vi "Test Process Cleared on Upstream Error.vi"(8 "error in (no error)":errorcluster, 11 "Process Test In":refnum<class "Process Dev Test.lvclass">) -> (0 "error out":errorcluster, 3 "Process Test Out":refnum<class "Process Dev Test.lvclass">)   [LabVIEW 2020, in "Process Dev Test.lvclass"]
uses:
  Process Dev Test.lvclass
  C:/Git/astemes-triarc-framework/source/TF Test Suite/Base Class Test/Base Test.lvclass
  C:/Program Files (x86)/National Instruments/LabVIEW 2020/vi.lib/Astemes/LUnit/Test Case.lvclass
  source/Framework/Process/Process.lvclass
  source/Framework/Process/Public/Lifecycle/Lifecycle State.ctl
  source/Framework Test Suite/Base Class Test/Base Test.lvclass/Base Test.ctl
  source/Framework/Process/Process.lvclass/Process.ctl
  <vilib>/Astemes/LUnit/Test Case.lvclass/Test Case.ctl
  <vilib>/Astemes/LUnit/LUnit Assertion Result.lvclass/LUnit Assertion Result.ctl
  <vilib>/Astemes/LUnit/LUnit Test Case Result.lvclass/LUnit Test Case Result.ctl
  <vilib>/Astemes/LUnit/LUnit Method Result.lvclass/LUnit Method Result.ctl
  <vilib>/Astemes/LUnit/Palette/Fail.vi
  <vilib>/Astemes/LUnit/Palette/Pass.vi
  <vilib>/Astemes/LUnit/Set Assertion Type.vi
  <vilib>/Astemes/LUnit/Add test result.vi
  <vilib>/Astemes/LUnit/LUnit Write Passed.vi
  <vilib>/Astemes/LUnit/LUnit Write Message.vi
  <vilib>/Astemes/LUnit/LUnit Write Description.vi
  <vilib>/Astemes/LUnit/LUnit Write Assertion Type.vi
  <vilib>/Astemes/LUnit/LUnit Record Assertion Result.vi
  <vilib>/Astemes/LUnit/LUnit Aggregate Assertion Results.vi
  <vilib>/Astemes/LUnit/Assertion Result/LUnit Read Status.vi
  <vilib>/Astemes/LUnit/LUnit Read Message.vi
  <vilib>/Astemes/LUnit/LUnit Read Description.vi
  <vilib>/Astemes/LUnit/Method Result/LUnit Merge Status.vi
  <vilib>/Astemes/LUnit/LUnit Concatenate result strings.vi
  source/Framework/Base/Base.lvclass
  <vilib>/Astemes/LUnit/LUnit Assertion Result.lvclass
  source/Framework Test Suite/Base Class Test/Base Test.lvclass
  <vilib>/Astemes/LUnit/Test Case.lvclass
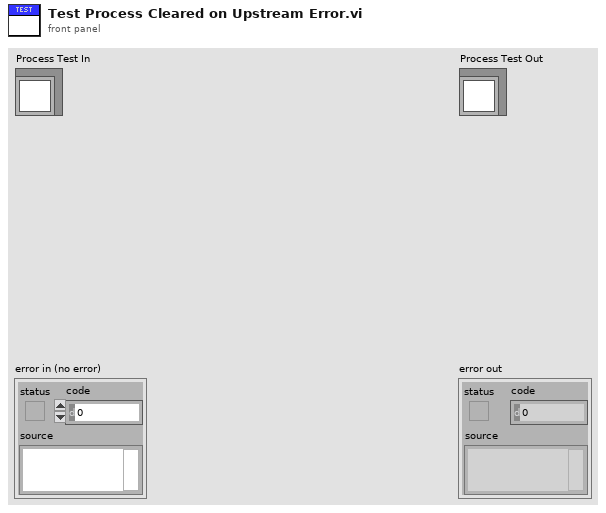
[diagram p1: front panel]
types:
  T1 = typedef "Process.lvclass/Lifecycle State.ctl" = enum16{"Uninitialized", "Initialized", "Started", "Running", "Stopped", "Finished"}
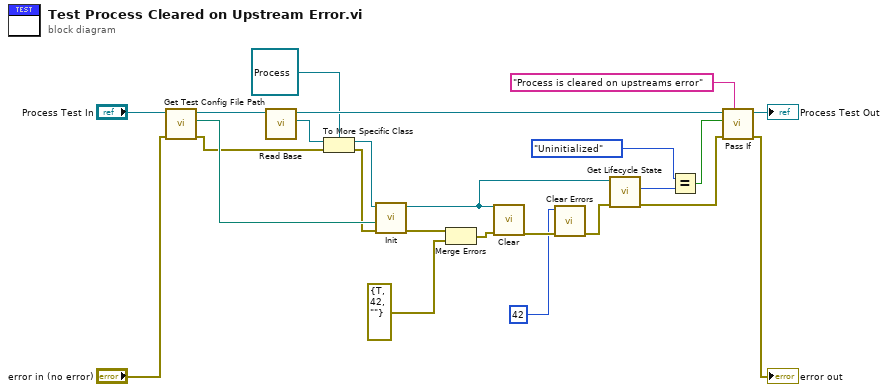
[diagram p0: block diagram]
diagram:
  n1 = call "Get Test Config File Path.vi"("error in (no error)"="error in (no error)", "Process Test In"="Process Test In") -> ("error out"=w14:errorcluster, "Test config path"=w20:path, "Process Test Out"=w22:refnum<class "Process Dev Test.lvclass">)  [unwired: 7 in]
  n2 = call "Read Base.vi"("Base Class Test In"=w22) -> ("Base.lvclass"=w17:refnum<class "Base.lvclass">, "Base Class Test Out"=w19:refnum<class "Process Dev Test.lvclass">)  [unwired: 8 in, 1 out]
  n3 = To More Specific Class(target class=refnum<class "Process.lvclass"> refnum ("Process.lvclass"), reference=w17, error in=w14) -> (specific class reference=w16:refnum<class "Process.lvclass">, error out=w15:errorcluster)
  n4 = call-dynamic "Init.vi"("error in (no error)"=w15, "Config File Path"=w20, "Process In"=w16) -> ("error out"=w23:errorcluster, "Process Out"=w1:refnum<class "Process.lvclass">)  [unwired: 7 in]
  n5 = Merge Errors(w23, errorcluster {"status"=TRUE, "code"=42, "source"=""} ("error constant")) -> (w3:errorcluster)
  n6 = call-dynamic "Clear.vi"("error in (no error)"=w3, "Process In"=w1) -> ("error out"=w7:errorcluster)  [unwired: 9 in]
  n7 = call <vilib>:"Clear Errors.vi"("error in (no error)"=w7, "specific error code to clear (0: all)"=42 ("code")) -> ("error out"=w6:errorcluster)  [unwired: 4 in, 1 out]
  n8 = call "Get Lifecycle State.vi"("error in (no error)"=w6, "Process In"=w1) -> ("error out"=w9:errorcluster, "Lifecycle State"=w11:T1)  [unwired: 6 in, 2 out]
  n9 = Equal?(x=Lifecycle_State."Uninitialized" ("Lifecycle State"), y=w11) -> (x = y?=w10:bool)
  n10 = call <vilib>:"Pass If.vi"("Description"="Process is cleared on upstreams error", "error in (no error)"=w9, "Pass?"=w10, "LUnit Test Case In"=w19) -> ("error out"=→"error out":errorcluster, "LUnit Test Case Out"=→"Process Test Out":refnum<class "Process Dev Test.lvclass">)  [unwired: 6 in]
